vi "Switch Initialize Test.vi"(0 "SWI Instrument Record":T4, 5 "Seq Count":i32, 9 "Test Parameters In":T5, 11 "error in (no error)":errorcluster) -> (3 "SWI Position":variant, 4 "SWI Instrument ID":string, 6 "Next Action":string, 10 "Test Parameters Out":T5, 14 "Driver Refs":T1, 15 "error out":errorcluster {"code" format="%.0x"})   [LabVIEW 2011]
uses:
  TypeDefs/Switch Test Parameters.ctl
  TypeDefs/Switch Stimulus Parameters.ctl
  TypeDefs/Switch Type.ctl
  TypeDefs/Switch Instrument Info.ctl
  server/database/Stations/Instruments/Instrument Record.ctl
  TypeDefs/Switch Driver Refs.ctl
  drivers/SWI/SWI Driver Ref.ctl
  drivers/PFE/PFE Driver Ref.ctl
  drivers/SWI/SWI Command.ctl
  drivers/PFE/PFE Command.ctl
  drivers/SWI/SWI Instrument Info.ctl
  drivers/PFE/PFE Instrument Info.ctl
  drivers/SWI/Kaelus/TypeDefs/Kaelus SWI Position.ctl
  PIM/BPIM Web Engine/LIB/MODULES/SW Module/SW Tx Positions.ctl
  PIM/BPIM Web Engine/LIB/MODULES/SW Module/SW Rx Positions.ctl
  drivers/SWI/Sea-Level/TypeDefs/Sea-Level SWI Position.ctl
  drivers/PFE/Kaelus/TypeDefs/Kaelus PFE Position.ctl
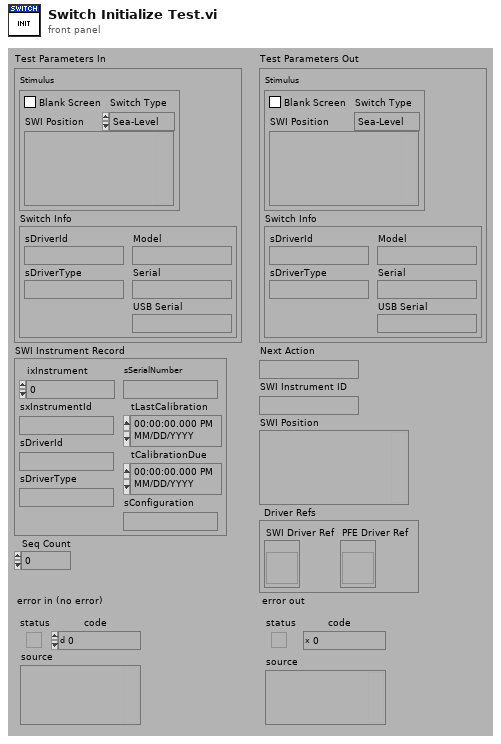
[diagram p1: front panel]
types:
  T1 = typedef "Switch Driver Refs.ctl" = cluster{"SWI Driver Ref":T2, "PFE Driver Ref":T3}
  T2 = typedef "SWI Driver Ref.ctl" = refnum<vi>
  T3 = typedef "PFE Driver Ref.ctl" = refnum<vi>
  T4 = typedef "Instrument Record.ctl" = cluster{"ixInstrument":i32, "sxInstrumentId":string, "sDriverId":string, "sDriverType":string, "sSerialNumber":string, "tLastCalibration":timestamp, "tCalibrationDue":timestamp, "sConfiguration":string}
  T5 = typedef "Switch Test Parameters.ctl" = cluster{"Stimulus":T6, "Switch Info":T8}
  T6 = typedef "Switch Stimulus Parameters.ctl" = cluster{"Blank Screen":bool, "SWI Position":variant, "Switch Type":T7}
  T7 = typedef "Switch Type.ctl" = enum16{"Sea-Level", "Simulator", "SI-0206-SW", "SI-0309-SW", "SI-0310-SW", "Front End"}
  T8 = typedef "Switch Instrument Info.ctl" = cluster{"sDriverId":string, "sDriverType":string, "Model":string, "Serial":string, "USB Serial":string}
  T9 = typedef "SWI Command.ctl" = enum16{"LOAD", "INITIALIZE", "PRESET", "SET STIMULUS", "GET STIMULUS", "GET INFO", "RELEASE", "UNLOAD"}
  T10 = typedef "PFE Command.ctl" = enum16{"LOAD", "INITIALIZE", "PRESET", "SET STIMULUS", "GET STIMULUS", "GET INFO", "RELEASE", "UNLOAD"}
  T11 = typedef "SWI Instrument Info.ctl" = cluster{"Model":string, "Serial":string, "USB Serial":string}
  T12 = typedef "PFE Instrument Info.ctl" = cluster{"Model":string, "Serial":string, "USB Serial":string}
  T13 = typedef "Kaelus SWI Position.ctl" = cluster{"Tx":T14, "Rx":T15}
  T14 = typedef "SW Tx Positions.ctl" = enum16{"TXA", "TXB", "TXC"}
  T15 = typedef "SW Rx Positions.ctl" = enum16{"RXA", "RXB", "RXC", "RXD", "RXE", "RXF"}
  T16 = typedef "Sea-Level SWI Position.ctl" = cluster{"Port 1 (0)":cluster{"0":bool, "1":bool, "2":bool, "3":bool, "4":bool, "5":bool, "6":bool, "7":bool}, "Port 2 (1)":cluster{"0":bool, "1":bool, "2":bool, "3":bool, "4":bool, "5":bool, "6":bool, "7":bool}, "Port 3 (2)":cluster{"0":bool, "1":bool, "2":bool, "3":bool, "4":bool, "5":bool, "6":bool, "7":bool}, "Port 4 (3)":cluster{"0":bool, "1":bool, "2":bool, "3":bool, "4":bool, "5":bool, "6":bool, "7":bool}}
  T17 = typedef "Kaelus PFE Position.ctl" = enum16{"P11 (P1 Reflected)", "P12 (P2 Through)", "P21 (P1 Through)", "P22 (P2 Reflected)"}
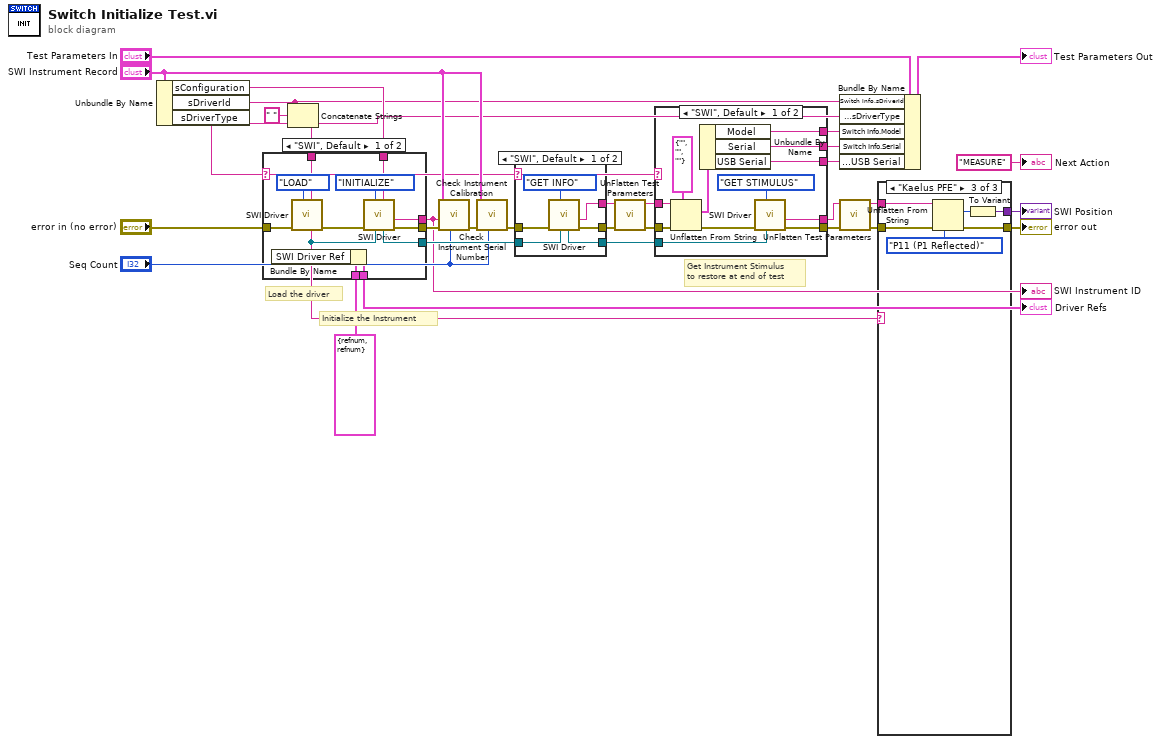
[diagram p0: block diagram]
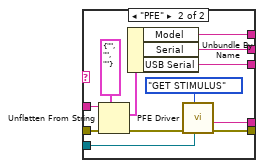
[diagram p2: hidden frame]
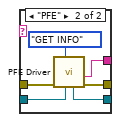
[diagram p3: hidden frame]
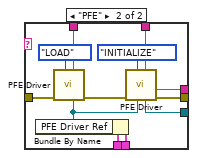
[diagram p4: hidden frame]
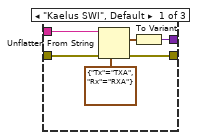
[diagram p5: hidden frame]
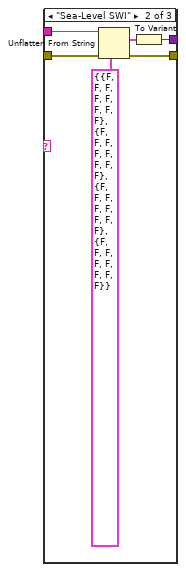
[diagram p6: hidden frame]
diagram:
  # "Get Instrument Stimulus\nto restore at end of test"
  # "Initialize the Instrument"
  # "Load the driver"
  n1 = Unbundle By Name("SWI Instrument Record") -> ("sConfiguration"=w32:string, "sDriverId"=w4:string, "sDriverType"=w6:string)
  n2 = Concatenate Strings(w4, " " ("string"), w6) -> (w3:string)
  n3 = case shown="\"SWI\", Default" w6 {
    tunnel: w32 -> [w44 w56]
    tunnel: w3 -> [w43 w55]
    tunnel: "error in (no error)" -> [w39 w51]
    tunnel: [w38 w50] -> w19
    tunnel: [w37 w49] -> w11
    tunnel: [w36 w48] -> w7
    tunnel: T1 {"SWI Driver Ref"=refnum, "PFE Driver Ref"=refnum} ("Driver Refs") -> [w35 w47]
    tunnel: [w33 w45] -> w1
    frame "SWI", Default {
      n4 = call "SWI Driver.vi"("SWI Configuration (\"\")"=w43, "SWI Command"=SWI_Command."LOAD", "error in (no error)"=w39) -> ("error out"=w40:errorcluster, "dup Drv Refnum"=w34:T2)  [unwired: 2 in, 5 out]
      n5 = Bundle By Name(cluster=w35, "SWI Driver Ref"=w34) -> (w33:T1)
      n6 = call "SWI Driver.vi"("SWI Configuration (\"\")"=w44, "Drv Refnum"=w34, "SWI Command"=SWI_Command."INITIALIZE", "error in (no error)"=w40) -> ("error out"=w37:errorcluster, "SWI Flat Output"=w36:string, "dup Drv Refnum"=w38:T2)  [unwired: 1 in, 4 out]
    }
    frame "PFE" {
      n7 = call "PFE Driver.vi"("PFE Configuration (\"\")"=w55, "PFE Command"=PFE_Command."LOAD", "error in (no error)"=w51) -> ("error out"=w52:errorcluster, "dup Drv Refnum"=w46:T3)  [unwired: 5 in, 2 out]
      n8 = Bundle By Name(cluster=w47, "PFE Driver Ref"=w46) -> (w45:T1)
      n9 = call "PFE Driver.vi"("PFE Configuration (\"\")"=w56, "Drv Refnum"=w46, "PFE Command"=PFE_Command."INITIALIZE", "error in (no error)"=w52) -> ("error out"=w49:errorcluster, "PFE Flat Output"=w48:string, "dup Drv Refnum"=w50:T3)  [unwired: 4 in, 1 out]
    }
  }
  "SWI Instrument ID" <- w7
  "Driver Refs" <- w1
  n10 = call "Check Instrument Serial Number.vi"("Seq Count"="Seq Count", "error in (no error)"=w11, "Instrument IDN String (\"\")"=w7, "Instrument Record"="SWI Instrument Record") -> ("error out"=w10:errorcluster)  [unwired: 7 out]
  n11 = call "Check Instrument Calibration.vi"("Seq Count"="Seq Count", "error in (no error)"=w10, "Instrument Record"="SWI Instrument Record") -> ("error out"=w20:errorcluster)  [unwired: 1 in, 7 out]
  n12 = case shown="\"SWI\", Default" w6 {
    tunnel: [w62 w68] -> w22
    tunnel: [w61 w67] -> w21
    tunnel: w20 -> [w59 w65]
    tunnel: w19 -> [w58 w64]
    tunnel: [w57 w63] -> w18
    frame "SWI", Default {
      n13 = call "SWI Driver.vi"("Drv Refnum"=w58, "SWI Command"=SWI_Command."GET INFO", "error in (no error)"=w59) -> ("error out"=w61:errorcluster, "SWI Flat Output"=w62:string, "dup Drv Refnum"=w57:T2)  [unwired: 2 in, 4 out]
    }
    frame "PFE" {
      n14 = call "PFE Driver.vi"("Drv Refnum"=w64, "PFE Command"=PFE_Command."GET INFO", "error in (no error)"=w65) -> ("error out"=w67:errorcluster, "PFE Flat Output"=w68:string, "dup Drv Refnum"=w63:T3)  [unwired: 5 in, 1 out]
    }
  }
  n15 = call "UnFlatten Test Parameters.vi"("error in (no error)"=w21, "Flattened Test Parameters with Version (\"\")"=w22) -> ("error out"=w16:errorcluster, "Flat Test Parameters"=w17:string)  [unwired: 4 out]
  n16 = case shown="\"SWI\", Default" w6 {
    tunnel: [w79 w91] -> w30
    tunnel: [w78 w90] -> w29
    tunnel: w18 -> [w77 w89]
    tunnel: w17 -> [w76 w88]
    tunnel: w16 -> [w75 w87]
    tunnel: [w71 w83] -> w13
    tunnel: [w70 w82] -> w12
    tunnel: [w69 w81] -> w5
    frame "SWI", Default {
      n17 = Unflatten From String(type=T11 {"Model"="", "Serial"="", "USB Serial"=""} ("SWI Information"), binary string=w76, error in (no error)=w75) -> (value=w72:T11, error out=w74:errorcluster)  [unwired: 3 out]
      n18 = Unbundle By Name(w72) -> ("Model"=w71:string, "Serial"=w70:string, "USB Serial"=w69:string)
      n19 = call "SWI Driver.vi"("Drv Refnum"=w77, "SWI Command"=SWI_Command."GET STIMULUS", "error in (no error)"=w74) -> ("error out"=w79:errorcluster, "SWI Flat Output"=w78:string)  [unwired: 2 in, 5 out]
    }
    frame "PFE" {
      n20 = Unflatten From String(type=T12 {"Model"="", "Serial"="", "USB Serial"=""} ("PFE Information"), binary string=w88, error in (no error)=w87) -> (value=w84:T12, error out=w86:errorcluster)  [unwired: 3 out]
      n21 = Unbundle By Name(w84) -> ("Model"=w83:string, "Serial"=w82:string, "USB Serial"=w81:string)
      n22 = call "PFE Driver.vi"("Drv Refnum"=w89, "PFE Command"=PFE_Command."GET STIMULUS", "error in (no error)"=w86) -> ("error out"=w91:errorcluster, "PFE Flat Output"=w90:string)  [unwired: 5 in, 2 out]
    }
  }
  n23 = Bundle By Name(cluster="Test Parameters In", "Switch Info.sDriverId"=w4, "Switch Info.sDriverType"=w6, "Switch Info.Model"=w13, "Switch Info.Serial"=w12, "Switch Info.USB Serial"=w5) -> (→"Test Parameters Out":T5)
  n24 = call "UnFlatten Test Parameters.vi"("error in (no error)"=w30, "Flattened Test Parameters with Version (\"\")"=w29) -> ("error out"=w27:errorcluster, "Flat Test Parameters"=w28:string)  [unwired: 4 out]
  n25 = case shown="\"Kaelus PFE\"" w3 {
    tunnel: w28 -> [w98 w104 w110]
    tunnel: w27 -> [w97 w103 w109]
    tunnel: [w96 w102 w108] -> w25
    tunnel: [w93 w99 w105] -> w23
    frame "Kaelus SWI", Default {
      n26 = Unflatten From String(type=T13 {"Tx"=enum."TXA", "Rx"=enum."RXA"} ("Switch Position"), binary string=w98, error in (no error)=w97) -> (value=w94:T13, error out=w96:errorcluster)  [unwired: 3 out]
      n27 = To Variant(anything=w94) -> (Variant=w93:variant)
    }
    frame "Sea-Level SWI" {
      n28 = Unflatten From String(type=T16 {"Port 1 (0)"={"0"=FALSE, "1"=FALSE, "2"=FALSE, "3"=FALSE, "4"=FALSE, "5"=FALSE, "6"=FALSE, "7"=FALSE}, "Port 2 (1)"={"0"=FALSE, "1"=FALSE, "2"=FALSE, "3"=FALSE, "4"=FALSE, "5"=FALSE, "6"=FALSE, "7"=FALSE}, "Port 3 (2)"={"0"=FALSE, "1"=FALSE, "2"=FALSE, "3"=FALSE, "4"=FALSE, "5"=FALSE, "6"=FALSE, "7"=FALSE}, "Port 4 (3)"={"0"=FALSE, "1"=FALSE, "2"=FALSE, "3"=FALSE, "4"=FALSE, "5"=FALSE, "6"=FALSE, "7"=FALSE}} ("SWI Stimulus"), binary string=w104, error in (no error)=w103) -> (value=w100:T16, error out=w102:errorcluster)  [unwired: 3 out]
      n29 = To Variant(anything=w100) -> (Variant=w99:variant)
    }
    frame "Kaelus PFE" {
      n30 = Unflatten From String(type=Kaelus_PFE_Position."P11 (P1 Reflected)" ("SWI Stimulus"), binary string=w110, error in (no error)=w109) -> (value=w106:T17, error out=w108:errorcluster)  [unwired: 3 out]
      n31 = To Variant(anything=w106) -> (Variant=w105:variant)
    }
  }
  "error out" <- w25
  "SWI Position" <- w23
  "Next Action" <- "MEASURE" ("Next Action")
